vi "AreWeInTransition.vi"() -> (3 "Boolean":bool)   [LabVIEW 2013]
doc: "This VI checks the past regime and checks whether we were in a transition. If so, the code will check whether the transistion has either failed or completed, and stays in transition otherwise. This is done to make sure a commanded transition goes to completion or failure instead rechecking every cycle whether the transition should be recommanded.\n\nEric Schneider, Feb. 2014"
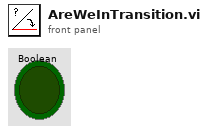
[diagram p1: front panel]
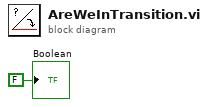
[diagram p0: block diagram]
diagram:
  "Boolean" <- FALSE ("Boolean")
